vi "Dereference-String.vi"(8 "No Error":errorcluster, 11 "Str [const char *]":i64 format="%.0x") -> (0 "error out":errorcluster, 3 "String":string)   [LabVIEW 2026, in "SDL3.lvlib" / "LV-Utilities.lvlib"]
doc: "<B>Summary</B>\nDereference <B>Str</B> pointer into <B>String</B>."
uses:
  LV-Utilities.lvlib
  Stdinc/Strlen.vi/c3f57b18-2899-4d18-8de7-ed42e0d99649.vi
  <vilib>/Utility/error.llb/Error Cluster From Error Code.vi
  Stdinc/Stdinc.lvlib
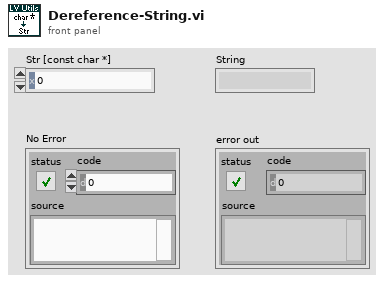
[diagram p1: front panel]
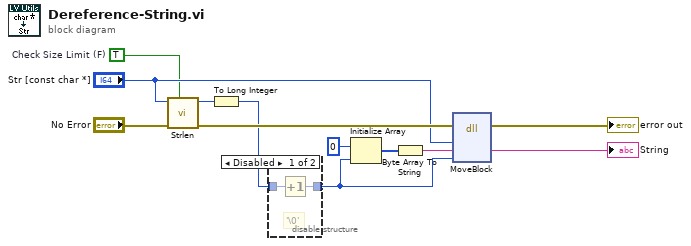
[diagram p0: block diagram]
diagram:
  w3 = TRUE  # Check Size Limit (F)
  n1 = call "Strlen.vi"("Check Size Limit (F)"=w3, "No Error"="No Error", "Str [const char *]"="Str [const char *]") -> ("Error Out"=w12:errorcluster, "Size"=w11:u64)  [unwired: 7 in]
  n2 = To Long Integer(number=w11) -> (32bit integer=w2:i32)
  n3 = disable-structure shown="Disabled" {
    disable-tunnel: [w14 w15] -> w7
    disable-tunnel: w2 -> [w13 w15]
    frame Disabled {
      # "'\\0'"
      n4 = Increment(x=w13) -> (x+1=w14:i32)
    }
    frame Enabled {
    }
  }
  n5 = Initialize Array(u8 0, w7) -> (w9:u8[])
  n6 = Byte Array To String(unsigned byte array=w9) -> (string=w8:string)
  n7 = dll-call lib="LabVIEW" fn="MoveBlock"(error in=w12, "Address"="Str [const char *]", "Destination"=w8, "Size"=w7) -> (error out=→"error out":errorcluster, "Destination"=→"String":string)  [unwired: 5 in, 1 out]
